vi "Handle.vi"(10 "log record":T1 {"timestamp" format="%<%x %.3X>T"}, 11 "handler in":refnum<class "Formatting Handler.lvclass">) -> (0 "writer error":errorcluster, 1 "formatter error":errorcluster, 3 "handler out":refnum<class "Formatting Handler.lvclass">)   [LabVIEW 2018, in "Logging.lvlib" / "Formatting Handler.lvclass"]
uses:
  Formatting Handler.lvclass
  Log Record.ctl
  logger_class/Internal Log Levels.ctl
  Formatting Handler.lvclass/Formatting Handler.ctl
  <vilib>/ErrorRing/Error Ring.xnode
  formatter_interface/Formatter.lvclass
  Logging.lvlib
panel:
  # "Connector Pane"
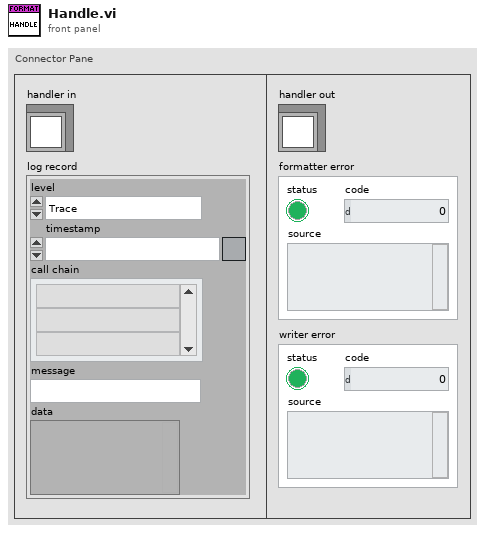
[diagram p1: front panel]
types:
  T1 = typedef "Logging.lvlib/Log Record.ctl" = cluster{"level":T2, "timestamp":timestamp, "call chain":string[], "message":string, "data":variant}
  T2 = typedef "Logging.lvlib/Internal Log Levels.ctl" = enum16{"Trace", "Debug", "Info", "Warning", "Error", "Critical", "Internal"}
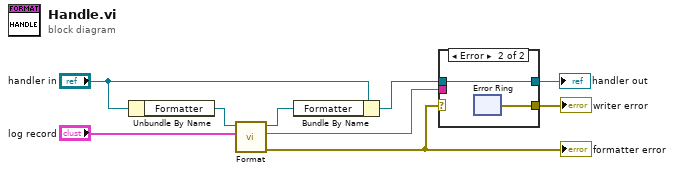
[diagram p0: block diagram]
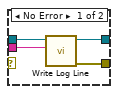
[diagram p2: hidden frame]
diagram:
  n1 = Unbundle By Name("handler in") -> ("Formatter"=w5:refnum<class "Formatter.lvclass">)
  n2 = call-dynamic "Format.vi"("log record"="log record", "formatter in"=w5) -> ("error out"=w1:errorcluster, "log line"=w2:string, "formatter out"=w4:refnum<class "Formatter.lvclass">)  [unwired: 7 in]
  "formatter error" <- w1
  n3 = Bundle By Name(cluster="handler in", "Formatter"=w4) -> (w3:refnum<class "Formatting Handler.lvclass">)
  n4 = case shown="Error" w1 {
    tunnel: [w13 w15] -> w9
    tunnel: [w12 w14] -> w6
    tunnel: w3 -> [w11 w15]
    tunnel: w2 -> [w10 _]
    frame No Error {
      n5 = call-dynamic "Write Log Line.vi"("log line"=w10, "handler in"=w11) -> ("error out"=w12:errorcluster, "handler out"=w13:refnum<class "Formatting Handler.lvclass">)  [unwired: 8 in]
    }
    frame Error {
      n6 = xnode "Error Ring"() -> ("error out"=w14:errorcluster)
    }
  }
  "handler out" <- w9
  "writer error" <- w6
